vi "Init-UserEventHandler.vi"(8 "error in":errorcluster, 9 "Level":T1, 10 "Name":string, 11 "UserEventHandler":refnum<class "UserEventHandler.lvclass">) -> (0 "error out":errorcluster, 3 "UserEventHandler out":refnum<class "UserEventHandler.lvclass">)   [LabVIEW 2020, in "hse-logger.lvlib" / "UserEventHandler.lvclass"]
doc: "Initiates a new ``UserEventHandler``-object with a name and log-level. This handler forwards the ``LogRecord`` to a User Event, a Event-Loop that has been registered for this event receives the ``LogRecord`` and can process it.\n\nThe handler forwards LogRecords only, if the level of the handler is greater or equal to the level of the LogRecord.\n\n____\nHAMPEL SOFTWARE ENGINEERING v2.0.6 (2021-04-15 11:38)"
uses:
  UserEventHandler.lvclass
  LogLevel.ctl
  LogRecord/LogRecord.lvclass
  UserEventHandler.lvclass/UserEventHandler.ctl
  hse-logger.lvlib
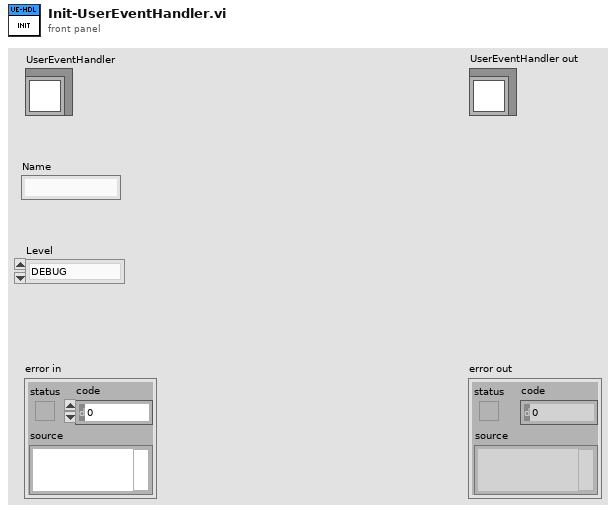
[diagram p1: front panel]
types:
  T1 = typedef "hse-logger.lvlib/LogLevel.ctl" = enum16{"DEBUG", "INFO", "WARNING", "ERROR", "CRITICAL"}
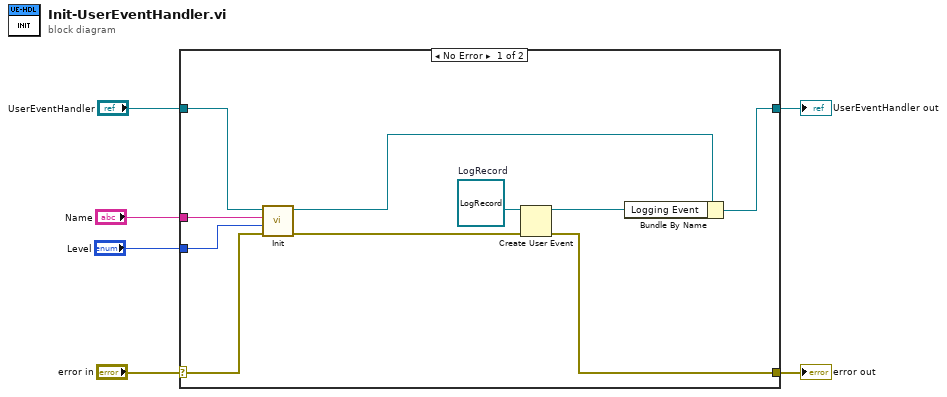
[diagram p0: block diagram]
diagram:
  n1 = case shown="No Error" "error in" {
    selector: "error in" -> [w16 w18]
    tunnel: [w14 w18] -> w5
    tunnel: [w11 w17] -> w4
    tunnel: "Name" -> [w9 _]
    tunnel: "Level" -> [w10 _]
    tunnel: "UserEventHandler" -> [w8 w17]
    frame No Error {
      w15 = refnum<class "LogRecord.lvclass"> refnum  # LogRecord
      n2 = call-dynamic "Init.vi"("error in"=w16, "Level"=w10, "Name"=w9, "Handler"=w8) -> ("error out"=w12:errorcluster, "Handler out"=w7:refnum<class "UserEventHandler.lvclass">)  [unwired: 6 in]
      n3 = Create User Event(user event datatype=w15, error in=w12) -> (user event=w13:refnum<user-event>, error out=w14:errorcluster)
      n4 = Bundle By Name(cluster=w7, "Logging Event"=w13) -> (w11:refnum<class "UserEventHandler.lvclass">)
    }
    frame Error {
    }
  }
  "error out" <- w5
  "UserEventHandler out" <- w4
